vi "Measure List Measurement.vi"(6 "Measurement":i32(ring) items=["None", "AC RMS", "Amplitude", "Average", "Cycle Average", "Cycle Frequency", "Cycle Period", "Cycle RMS", "DC RMS", "Estimated Number of Bits", "Falling Edges", "Fall Overshoot", "Fall Preshoot", "Frequency", "Fall Crossing Time", "Fall Time", "High", "Low", "Maximum", "Minimum", "Mid", "Negative Duty", "Negative Width", "Positive Duty", "Period", "Phase", "Peak to Peak", "Positive Width", "Rising Edges", "Rise Overshoot", "Rise Preshoot", "Rise Crossing Time", "Rise Time", "Standard Deviation", "Spurious Free Dynamic Range", "Signal to Noise+Distortion", "Signal to Noise", "Total Harmonic Distortion", "Time of Maximum", "Time of Minimum"], 7 "Source":i32(ring) items=["Input Channel 1", "Input Channel 2", "Input Channel 3", "Input Channel 4", "Calc Channel 1", "Calc Channel 2", "Calc Channel 3", "Calc Channel 4", "Ref Channel 1", "Ref Channel 2", "Ref Channel 3", "Ref Channel 4"], 8 "error in":errorcluster, 9 "Meas Number":i32(ring) caption="Measurement Number" items=["Measurement 1", "Measurement 2", "Measurement 3", "Measurement 4", "Measurement 5", "Measurement 6", "Measurement 7", "Measurement 8"], 10 "List Number":i32(ring) items=["List 1", "List 2", "List 3", "List 4"], 11 "Instrument Handle In":i32) -> (0 "error out":errorcluster, 3 "Instrument Handle Out":i32)   [LabVIEW 8.6, in "ZTScopeM.lvlib"]
doc: "This function sets the parameters for an individual measurement within a measurement set. There are 4 sets of 8 measurements each."
uses:
  ZTScopeM.lvlib
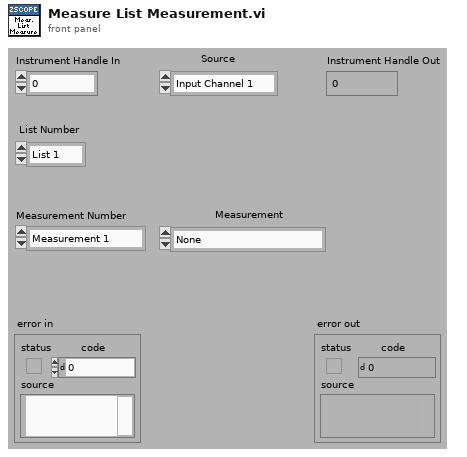
[diagram p1: front panel]
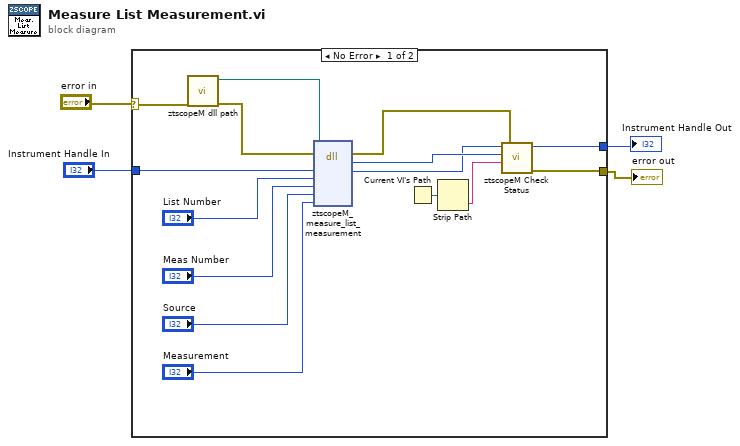
[diagram p0: block diagram]
diagram:
  n1 = case shown="No Error" "error in" {
    selector: "error in" -> [w8 w21]
    tunnel: [w10 w21] -> w1
    tunnel: "Instrument Handle In" -> [w19 w20]
    tunnel: [w9 w20] -> w3
    frame #0 {
      n2 = call "ztscopeM dll path.vi"("error in (no error)"=w8) -> ("error out"=w6:errorcluster, "<instrument>.dll path"=w7:path)  [unwired: 9 in]
      n3 = dll-call lib="C:/Program Files (x86)/National Instruments/LabVIEW 2013/instr.lib/ztscopem/ztscopeM.dll" fn="ztscopeM_measure_list_measurement"(path in=w7, error in=w6, "instrumentHandle"=w19, "listNumber"="List Number", "measurementNumber"="Meas Number", "source"="Source", "Measurement"="Measurement") -> (error out=w5:errorcluster, w12:i32, "instrumentHandle"=w11:i32)  [unwired: 5 in, 1 out]
      n4 = Current VI's Path() -> (path=w14:path)
      n5 = Strip Path(path=w14) -> (name=w13:string)  [unwired: 1 out]
      n6 = call "ztscopeM Check Status.vi"("error in"=w5, "name of VI"=w13, "status (return code)"=w12, "instrument handle in"=w11) -> ("error out"=w10:errorcluster, "instrument handle out"=w9:i32)  [unwired: 2 in]
    }
    frame #1 {
    }
  }
  "Instrument Handle Out" <- w3
  "error out" <- w1
